vi "Get Sentran Accuracy Test Settings.vi"(11 "Model in":refnum<class "Model.lvclass">) -> (2 "Sentran Accuracy Test Settings":T1 {"Max Moment (NM)" format="%.4f"; "Sample Time (s)" format="%.4f"; "Process Time (s)" format="%.4f"; "Force Tolerance (N)" format="%.4f"}, 3 "Model out":refnum<class "Model.lvclass">)   [LabVIEW 2016]
uses:
  Model.lvclass
  Typedefs/SentranAccuracyTestSettings.ctl
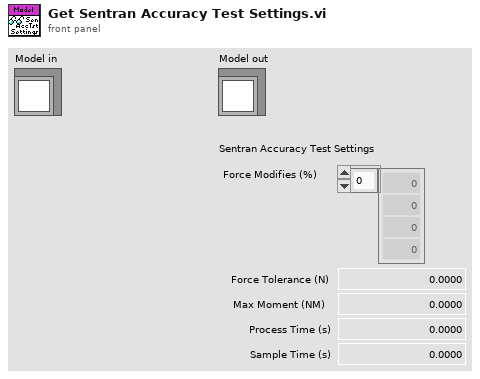
[diagram p1: front panel]
types:
  T1 = typedef "SentranAccuracyTestSettings.ctl" = cluster{"Force Tolerance (N)":dbl, "Force Modifies (%)":dbl[], "Process Time (s)":dbl, "Sample Time (s)":dbl, "Max Moment (NM)":dbl}
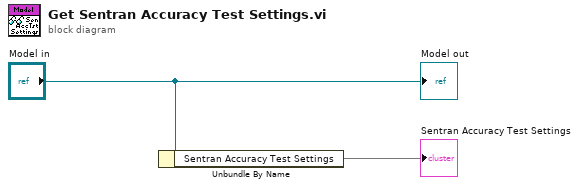
[diagram p0: block diagram]
diagram:
  n1 = Unbundle By Name("Model in") -> ("Sentran Accuracy Test Settings"=→"Sentran Accuracy Test Settings")
  "Model out" <- "Model in"
